vi "Set NrOfTXPDO.vi"(10 "NrOfTXPDO":u16, 11 "Device Info in":refnum<class "Device Info.lvclass">) -> (3 "Device Info out":refnum<class "Device Info.lvclass">)   [LabVIEW 2024, in "EDS.lvlib" / "Device Info.lvclass"]
uses:
  Device Info.lvclass
  Device Info.lvclass/Device Info.ctl
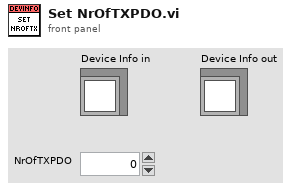
[diagram p1: front panel]
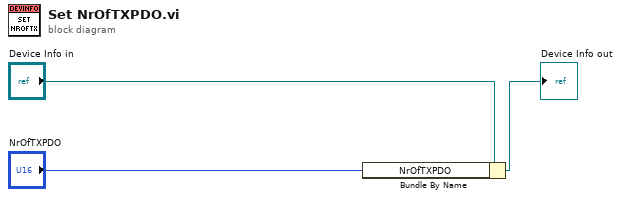
[diagram p0: block diagram]
diagram:
  n1 = Bundle By Name(cluster="Device Info in", "NrOfTXPDO"="NrOfTXPDO") -> (→"Device Info out":refnum<class "Device Info.lvclass">)
